vi "test.vi"(1 "Image":T1, 7 "error in":errorcluster) -> (20 "Matches (Geometric Matching 1)":T2[](array[typedef]) {"Correlation Score" format="%.2f"; "Target Template Curve Score" format="%.2f"; "Template Target Curve Score" format="%.2f"; "Bounding Box"."y" format="%.2f"; "Bounding Box"."x" format="%.2f"; "Position"."y" format="%.2f"; "Position"."x" format="%.2f"; "Score" format="%.2f"; "Scale" format="%.2f"; "Angle" format="%.2f"; "Occlusion %" format="%.2f"}, 21 "Calibrated Matches (Geometric Matching 1)":T2[](array[typedef]) {"Correlation Score" format="%.2f"; "Target Template Curve Score" format="%.2f"; "Template Target Curve Score" format="%.2f"; "Bounding Box"."y" format="%.2f"; "Bounding Box"."x" format="%.2f"; "Position"."y" format="%.2f"; "Position"."x" format="%.2f"; "Score" format="%.2f"; "Scale" format="%.2f"; "Angle" format="%.2f"; "Occlusion %" format="%.2f"}, 22 "Number of Matches (Geometric Matching 1)":i32, 23 "Image Out":T1(plugin-control), 27 "error out":errorcluster)   [LabVIEW 2016]
uses:
  <vilib>/vision/Pattern Matching.llb/IMAQ GM Match Report.ctl
  <vilib>/vision/Image Controls.llb/IMAQ Image.ctl
  <vilib>/vision/Pattern Matching.llb/IMAQ Curve Parameters.ctl
  <vilib>/vision/Pattern Matching.llb/IMAQ Match Range Setting.ctl
  <vilib>/vision/NI_Vision_Development_Module.lvlib
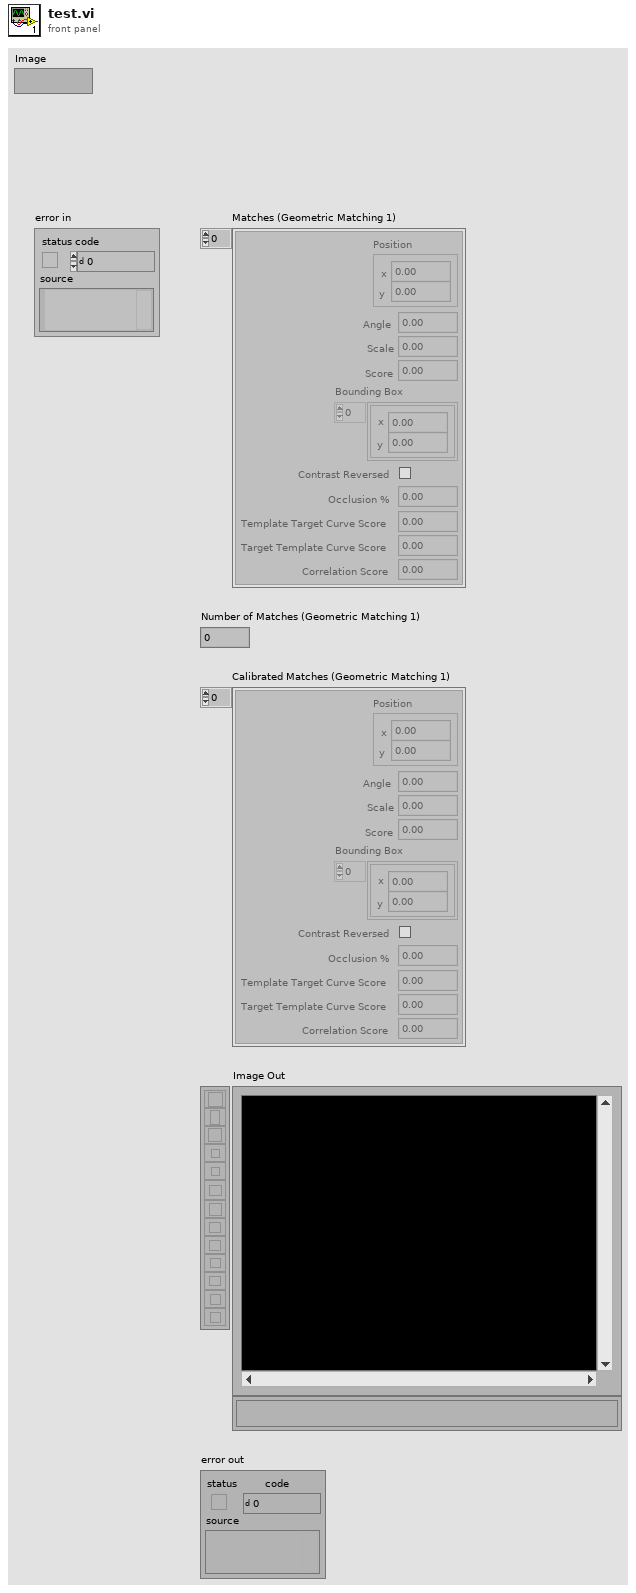
[diagram p1: front panel]
types:
  T1 = typedef "IMAQ Image.ctl" = refnum<image>
  T2 = typedef "IMAQ GM Match Report.ctl" = cluster{"Position":cluster{"x":sgl, "y":sgl}, "Angle":sgl, "Scale":sgl, "Score":sgl, "Bounding Box":cluster{"x":sgl, "y":sgl}[], "Contrast Reversed":bool, "Occlusion %":sgl, "Template Target Curve Score":sgl, "Target Template Curve Score":sgl, "Correlation Score":sgl}
  T3 = typedef "IMAQ Curve Parameters.ctl" = cluster{"Extraction Mode":u32, "Edge Threshold":i32, "Edge Filter Size":u32, "Min Length":i32, "Row Search Step Size":i32, "Col Search Step Size":i32, "Max Endpoint Gap":i32, "Closed":bool, "Subpixel":bool}
  T4 = typedef "IMAQ Match Range Setting.ctl" = cluster{"Match Constraints":u32, "Min":dbl, "Max":dbl}
  T5 = cluster{"Curve Parameters":T3, "Match Mode":cluster{"Rotation":bool, "Scale":bool, "Occlusion":bool, "Reserved":bool, "Reserved":bool, "Reserved":bool}, "Range Settings":T4[], "Number of Matches":i32, "Minimum Match Score":sgl, "SubPixel Accuracy":bool, "Adv. Geometric Match Options 2":cluster{"Setup Data Item":u16, "Item Value":dbl}[]}
  T6 = cluster{"Global Rectangle":i32[], "Contours":cluster{"ID":enum32{"External", "Internal"}, "Type":u32, "Coordinates":i32[]}[]}
  T7 = cluster{"Brightness":sgl, "Contrast":sgl, "Gamma":sgl}
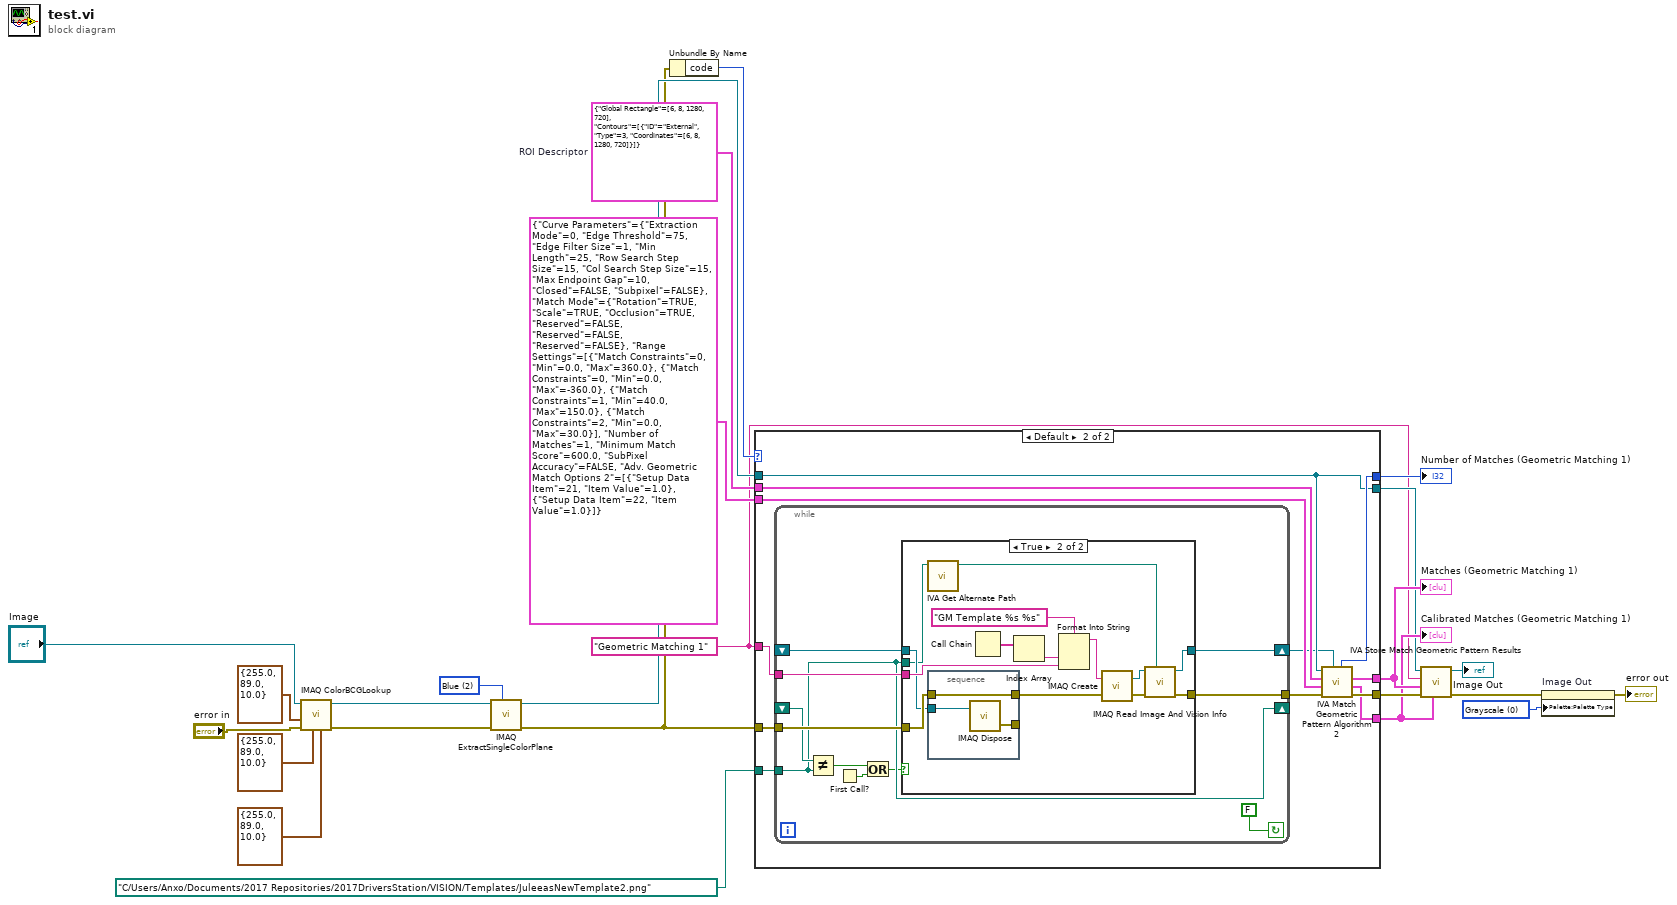
[diagram p0: block diagram]
diagram:
  w3 = u32 0 items=["Grayscale", "Binary", "Gradient", "Rainbow", "Temperature", "User Defined", "Binary 16 Bit", "Gradient 16 Bit", "Rainbow 16 Bit", "Temperature 16 Bit", "User Defined 16 Bit"] ("Palette Type")
  w7 = "Geometric Matching 1" ("Step Name")
  w17 = T6 {"Global Rectangle"=[6, 8, 1280, 720], "Contours"=[{"ID"=enum."External", "Type"=3, "Coordinates"=[6, 8, 1280, 720]}]}  # ROI Descriptor
  w21 = 2 items=["Red", "Green", "Blue", "Hue", "Saturation", "Luminance", "Value", "Intensity"] ("Color Plane")
  n1 = call "IMAQ ColorBCGLookup"("Blue BCG Values"=T7 {"Brightness"=255.0, "Contrast"=89.0, "Gamma"=10.0}, "Green BCG Values"=T7 {"Brightness"=255.0, "Contrast"=89.0, "Gamma"=10.0}, "error in (no error)"="error in", "Red BCG Values"=T7 {"Brightness"=255.0, "Contrast"=89.0, "Gamma"=10.0}, "Image Src"="Image") -> ("error out"=w19:errorcluster, "Image Dst Out"=w20:T1)  [unwired: 2 in, 3 out]
  n2 = call "IMAQ ExtractSingleColorPlane"("Color Plane"=w21, "error in (no error)"=w19, "Image Src"=w20) -> ("error out"=w11:errorcluster, "Image Dst Out"=w16:T1)  [unwired: 1 in, 6 out]
  n3 = Unbundle By Name(w11) -> ("code"=w10:i32)
  n4 = case shown="Default" w10 {
    tunnel: path "C:/Users/Anxo/Documents/2017 Repositories/2017DriversStation/VISION/Templates/JuleeasNewTemplate2.png" ("Template File Path") -> [_ w30]
    tunnel: w11 -> [_ w29]
    tunnel: T5 {"Curve Parameters"={"Extraction Mode"=0, "Edge Threshold"=75, "Edge Filter Size"=1, "Min Length"=25, "Row Search Step Size"=15, "Col Search Step Size"=15, "Max Endpoint Gap"=10, "Closed"=FALSE, "Subpixel"=FALSE}, "Match Mode"={"Rotation"=TRUE, "Scale"=TRUE, "Occlusion"=TRUE, "Reserved"=FALSE, "Reserved"=FALSE, "Reserved"=FALSE}, "Range Settings"=[{"Match Constraints"=0, "Min"=0.0, "Max"=360.0}, {"Match Constraints"=0, "Min"=0.0, "Max"=-360.0}, {"Match Constraints"=1, "Min"=40.0, "Max"=150.0}, {"Match Constraints"=2, "Min"=0.0, "Max"=30.0}], "Number of Matches"=1, "Minimum Match Score"=600.0, "SubPixel Accuracy"=FALSE, "Adv. Geometric Match Options 2"=[{"Setup Data Item"=21, "Item Value"=1.0}, {"Setup Data Item"=22, "Item Value"=1.0}]} ("Settings") -> [_ w37]
    tunnel: w17 -> [_ w36]
    tunnel: w16 -> [w25 w31]
    tunnel: [_ w35] -> w15
    tunnel: [_ w34] -> w14
    tunnel: [_ w33] -> w13
    tunnel: [_ w32] -> w12
    tunnel: [w25 w31] -> w9
    tunnel: w7 -> [_ w26]
    frame -1074396199, -1074396198 {
      # "Discard Coordinate System Error"
    }
    frame Default {
      n5 = while {
        shift-right: [w48] -> w27
        shift-left: _ -> [w47]
        tunnel: [w45] -> w28
        tunnel: w29 -> [w44]
        tunnel: w30 -> [w41]
        tunnel: w26 -> [w43]
        shift-right: [w41] -> _
        shift-left: _ -> [w42]
        stop <- FALSE continue-if-true
        n6 = Not Equal?(x=w42, y=w41) -> (x != y?=w39:bool)
        n7 = First Call?() -> (First Call?: T/F=w40:bool)
        n8 = Or(x=w39, y=w40) -> (x .or. y?=w38:bool)
        n9 = case shown="True" w38 {
          tunnel: [w50 w62] -> w48
          tunnel: w47 -> [w50 w54]
          tunnel: [w49 w59] -> w45
          tunnel: w44 -> [w49 w55]
          tunnel: w43 -> [_ w56]
          tunnel: w41 -> [_ w52]
          frame False {
          }
          frame True {
            n10 = call <vilib>:"IVA Get Alternate Path.vi"("Path In"=w52) -> ("Path Out"=w51:path)  [unwired: 10 out]
            n11 = stacked-sequence {
              tunnel: w55 -> [w67]
              tunnel: w54 -> [w66]
              tunnel: [w67] -> w53
              tunnel: [w65] -> _
              frame #0 {
                n12 = call "IMAQ Dispose"("Image"=w66) -> ("error out"=w65:errorcluster)  [unwired: 2 in, 3 out]
              }
            }
            n13 = Call Chain() -> (call chain=w58:string[])
            n14 = Index Array(array=w58) -> (element=w57:string)  [unwired: 1 in]
            n15 = Format Into String(format string="GM Template %s %s" ("Image Name"), w57, w56) -> (resulting string=w64:string)  [unwired: 2 in, 1 out]
            n16 = call "IMAQ Create"("Image Name"=w64, "error in (no error)"=w53) -> ("New Image"=w61:T1, "error out"=w60:errorcluster)  [unwired: 2 in, 1 out]
            n17 = call "IMAQ Read Image And Vision Info"("File Path"=w51, "error in (no error)"=w60, "Image"=w61) -> ("error out"=w59:errorcluster, "Image Out"=w62:T1)  [unwired: 1 in, 6 out]
          }
        }
      }
      n18 = call <vilib>:"IVA Match Geometric Pattern Algorithm 2.vi"("Template"=w27, "error in (no error)"=w28, "Settings"=w37, "ROI Descriptor"=w36, "Image"=w31) -> ("error out"=w35:errorcluster, "Calibrated Matches"=w33:T2[], "Matches"=w34:T2[], "Number of Matches"=w32:i32)  [unwired: 1 in, 2 out]
    }
  }
  "Matches (Geometric Matching 1)" <- w14
  "Number of Matches (Geometric Matching 1)" <- w12
  "Calibrated Matches (Geometric Matching 1)" <- w13
  n19 = call <vilib>:"IVA Store Match Geometric Pattern Results.vi"("Calibrated Matches"=w13, "error in (no error)"=w15, "Matches"=w14, "Step Name"=w7, "Image in"=w9) -> ("error out"=w6:errorcluster, "Image dup"=→"Image Out":T1)  [unwired: 5 out]
  n20 = property on="Image Out" class="ImageControl"(error in=w6, "Palette:Palette Type"=w3) -> (error out=→"error out":errorcluster)  [unwired: 1 in, 1 out]
